vi "PCert-DiscoverActors.vi"(7 "Custom Config Pages Directory":path, 11 "error in":errorcluster) -> (4 "Configuration Actor Filepaths":path[](array[path]), 6 "Display Names":string[](array[string]), 8 "Descriptions":string[](array[string]), 10 "Tree Tags":string[](array[string]), 15 "error out":errorcluster)   [LabVIEW 2013, in "PCert-Container-UI.lvclass"]
uses:
  PCert-Container-UI.lvclass
  ERP-ActorPlugins/Plugins/ActorPlugin-001-CreateInstructions.vi
  ERP-ActorPlugins/Plugins/ActorPlugin-002-Inventory.vi
  ERP-ActorPlugins/Plugins/ActorPlugin-003-CreateWorkOrder.vi
  Actors/ERP-Create Instructions Plugin/ERP-CreateInstructions/ERP-CreateInstructions.lvclass
  Actors/ERP-Inventory Plugin/ERP-Inventory.lvclass
  Actors/ERP-Create Work Order/ERP-CreateWorkOrder.lvclass
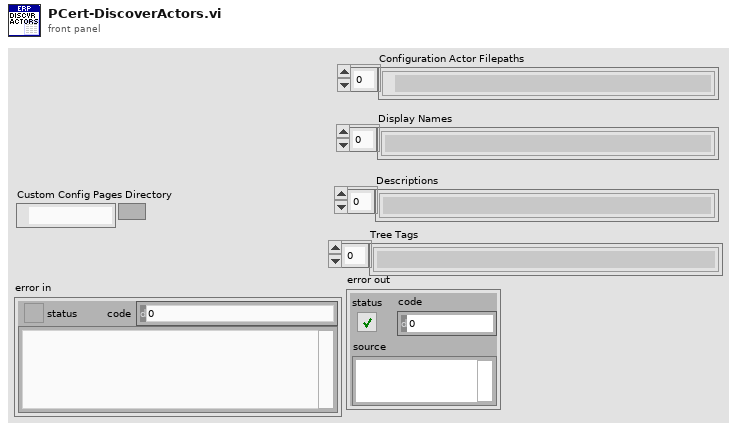
[diagram p1: front panel]
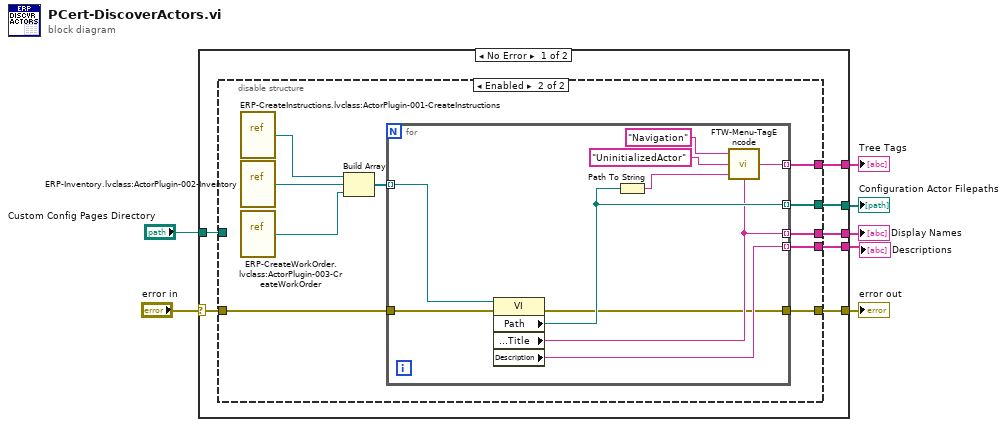
[diagram p0: block diagram]
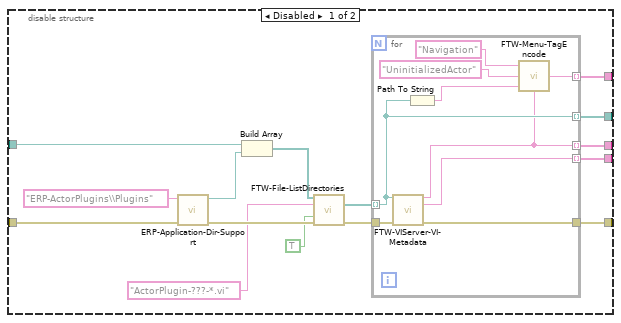
[diagram p2: hidden frame]
diagram:
  n1 = case shown="No Error" "error in" {
    selector: "error in" -> [w14 w59]
    tunnel: "Custom Config Pages Directory" -> [w13 _]
    tunnel: [w12 _] -> w5
    tunnel: [w11 _] -> w4
    tunnel: [w10 _] -> w3
    tunnel: [w9 w59] -> w2
    tunnel: [w8 _] -> w1
    frame No Error {
      n2 = disable-structure shown="Enabled" {
        disable-tunnel: w14 -> [w26 w40]
        disable-tunnel: w13 -> [w25 _]
        disable-tunnel: [w19 w48] -> w12
        disable-tunnel: [w18 w47] -> w11
        disable-tunnel: [w17 w46] -> w10
        disable-tunnel: [w16 w45] -> w9
        disable-tunnel: [w15 w44] -> w8
        frame Disabled {
          n3 = call "ERP-Application-Dir-Support.vi"("error in"=w26, "Support Resource Relative Filepath"="ERP-ActorPlugins\\Plugins") -> ("error out"=w29:errorcluster, "Support Path"=w28:path)  [unwired: 8 in]
          n4 = Build Array(w25, w28) -> (w24:path[])
          n5 = call "FTW-File-ListDirectories.vi"("Directories"=w24, "Matching Filename Pattern"="ActorPlugin-???-*.vi" ("Support Resource Relative Filepath"), "Treat LLBs as Folders?"=TRUE, "error in"=w29) -> ("Matching Filepaths"=w21:path[], "error out"=w20:errorcluster)  [unwired: 9 in, 1 out]
          n6 = for {
            tunnel: w21 -> [w31] mode=indexing
            tunnel: w20 -> [w38]
            tunnel: [w30] -> w18 mode=indexing
            tunnel: [w37] -> w17 mode=indexing
            tunnel: [w36] -> w16
            tunnel: [w32] -> w19 mode=indexing
            tunnel: [w31] -> w15 mode=indexing
            n7 = call "FTW-VIServer-VI-Metadata.vi"("VI Filepath"=w31, "error in"=w38) -> ("Front Panel Title"=w30:string, "VI Description"=w37:string, "error out"=w36:errorcluster)  [unwired: 11 in]
            n8 = Path To String(path=w31) -> (string=w35:string)
            n9 = call "FTW-Menu-TagEncode.vi"("Actor Name"=w30, "Payload"=w35, "Command"="UninitializedActor", "Class"="Navigation") -> ("Tag"=w32:string)
          }
        }
        frame Enabled {
          n10 = vi-ref "ERP-CreateInstructions.lvclass:ActorPlugin-001-CreateInstructions.vi"() -> (w43:refnum<vi>)
          n11 = vi-ref "ERP-Inventory.lvclass:ActorPlugin-002-Inventory.vi"() -> (w42:refnum<vi>)
          n12 = vi-ref "ERP-CreateWorkOrder.lvclass:ActorPlugin-003-CreateWorkOrder.vi"() -> (w39:refnum<vi>)
          n13 = Build Array(w43, w42, w39) -> (w41:refnum<vi>[])
          n14 = for {
            tunnel: [w52] -> w47 mode=indexing
            tunnel: [w51] -> w46 mode=indexing
            tunnel: [w49] -> w45
            tunnel: [w55] -> w48 mode=indexing
            tunnel: [w53] -> w44 mode=indexing
            tunnel: w41 -> [w54] mode=indexing
            tunnel: w40 -> [w50]
            n15 = property class="VI"(reference=w54, error in=w50) -> (error out=w49:errorcluster, "Path"=w53:path, "Front Panel.Title"=w52:string, "Description"=w51:string)  [unwired: 1 out]
            n16 = Path To String(path=w53) -> (string=w58:string)
            n17 = call "FTW-Menu-TagEncode.vi"("Actor Name"=w52, "Payload"=w58, "Command"="UninitializedActor", "Class"="Navigation") -> ("Tag"=w55:string)
          }
        }
      }
    }
    frame Error {
    }
  }
  "Tree Tags" <- w5
  "Display Names" <- w4
  "Descriptions" <- w3
  "error out" <- w2
  "Configuration Actor Filepaths" <- w1
